vi "Check.vi"(4 "Encoding":T2, 6 "Type":T3, 7 "Port":i32=22, 8 "Error In":errorcluster, 9 "Host Key":u8[](array[numeric]), 10 "Address":string, 11 "KnownHosts In":refnum<class "Known Hosts.lvclass">) -> (0 "Error Out":errorcluster, 2 "Result":T1, 3 "KnownHosts Out":refnum<class "Known Hosts.lvclass">)   [LabVIEW 2018, in "Toolkit.lvlib" / "Known Hosts.lvclass"]
uses:
  Known Hosts.lvclass
  Typedefs/Host Name Types.ctl
  Typedefs/Key Encodings.ctl
  Typedefs/Check Results.ctl
  Known Hosts.lvclass/Known Hosts.ctl
  Session/Session.lvclass/Session.ctl
  SSH/SSH.lvclass/SSH.ctl
  Toolkit.lvlib
  Session/Session.lvclass
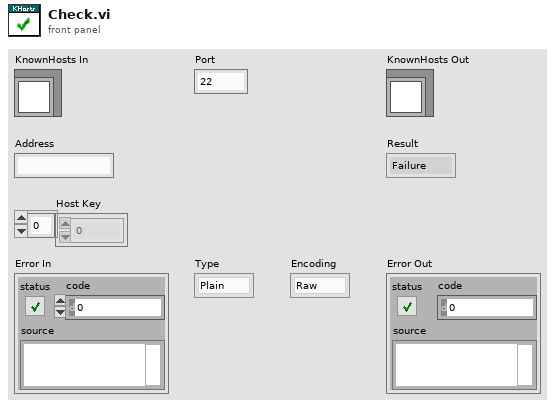
[diagram p1: front panel]
types:
  T1 = typedef "Toolkit.lvlib/Known Hosts.lvclass/Check Results.ctl" = enum32{"Failure", "Mismatch", "Match", "Not Found"}
  T2 = typedef "Toolkit.lvlib/Known Hosts.lvclass/Key Encodings.ctl" = enum32{"Raw", "Base64"}
  T3 = typedef "Toolkit.lvlib/Known Hosts.lvclass/Host Name Types.ctl" = enum32{"Plain", "SHA1", "Custom"}
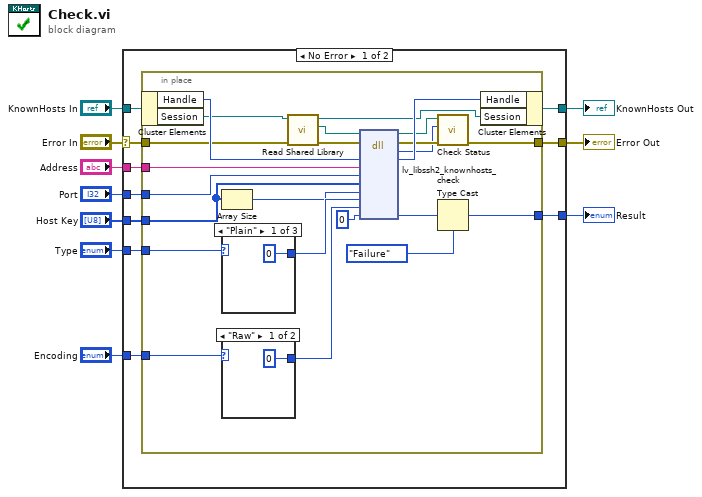
[diagram p0: block diagram]
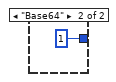
[diagram p2: hidden frame]
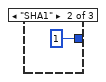
[diagram p3: hidden frame]
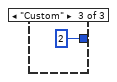
[diagram p4: hidden frame]
diagram:
  n1 = case shown="No Error" "Error In" {
    selector: "Error In" -> [w18 w50]
    tunnel: "KnownHosts In" -> [w20 w49]
    tunnel: [w17 w50] -> w8
    tunnel: [w19 w49] -> w7
    tunnel: "Address" -> [w16 _]
    tunnel: "Host Key" -> [w15 _]
    tunnel: "Type" -> [w14 _]
    tunnel: "Encoding" -> [w13 _]
    tunnel: "Port" -> [w12 _]
    tunnel: [w11 _] -> w1
    frame No Error {
      n2 = in-place {
        in-place-border: w18 -> [w38]
        in-place-border: [w37] -> w17
        in-place-border: w16 -> [w39]
        in-place-border: w15 -> [w30]
        in-place-border: w14 -> [w35]
        in-place-border: w13 -> [w33]
        in-place-border: w12 -> [w31]
        in-place-border: [w25] -> w11
        n3 = in-place-cluster #1(w20) -> ("Handle"=w43:u64, "Session"=w23:refnum<class "Session.lvclass">)
        n4 = Array Size(array=w30) -> (size(s)=w29:i32)
        n5 = case shown="\"Plain\"" w35 {
          tunnel: [0 1 2] -> w34
          frame "Plain" {
          }
          frame "SHA1" {
          }
          frame "Custom" {
          }
        }
        n6 = case shown="\"Raw\"" w33 {
          tunnel: [0 1] -> w32
          frame "Raw" {
          }
          frame "Base64" {
          }
        }
        n7 = call "Read Shared Library.vi"("Error In"=w38, "Session In"=w23) -> ("Erorr Out"=w24:errorcluster, "libssh2lv Shared Library"=w22:path, "Session Out"=w21:refnum<class "Session.lvclass">)  [unwired: 7 in]
        n8 = dll-call lib="D:/Users/cfield/Code/Field R&D Services/SSH/LV-LIBSSH2/LabVIEW/trunk/src/Toolkit/Support/lv-libssh2.*" fn="lv_libssh2_knownhosts_check"(path in=w22, error in=w24, "handle"=w43, "host"=w39, "port"=w31, "host_key"=w30, "host_key_len"=w29, "type"=w34, "encoding"=w32, "result"=0) -> (path out=w40:path, error out=w41:errorcluster, "status"=w36:i32, "handle"=w42:u64, "result"=w27:i32)  [unwired: 7 in]
        n9 = call "Check Status.vi"("Error In"=w41, "Status"=w36, "lv-libssh2 Shared Library In"=w40) -> ("Error Out"=w37:errorcluster)  [unwired: 7 in, 1 out]
        n10 = Type Cast(type=Check_Results."Failure" ("Result"), x=w27) -> (*(type *) &x=w25:T1)
        n11 = in-place-cluster #1("Handle"=w42, "Session"=w21) -> (w19:refnum<class "Known Hosts.lvclass">)
      }
    }
    frame Error {
    }
  }
  "Error Out" <- w8
  "KnownHosts Out" <- w7
  "Result" <- w1
